vi "Module Type.vi"(11 "Historian Logger in":refnum<class "Historian Logger.lvclass">) -> (2 "Module Type":string)   [LabVIEW 2020, in "VolatusHistorian.lvlib" / "Historian Logger.lvclass"]
uses:
  Historian Logger.lvclass
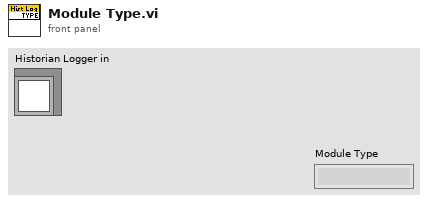
[diagram p1: front panel]
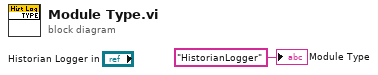
[diagram p0: block diagram]
diagram:
  "Module Type" <- "HistorianLogger" ("Module Type")
